vi "Get UUT Error.vi"(8 "error in (no error)":errorcluster, 11 "VISA resource name":refnum<visa-resource-name>) -> (0 "error out":errorcluster, 1 "Error Units":i32, 2 "Value of Error":dbl format="%.4f", 3 "VISA resource name out":refnum<visa-resource-name>)   [LabVIEW 2011, in "Fluke 5XXX Series Multicalibrators.lvlib"]
doc: "This VI returns the UUT error and units computed by the Calibrator after shifting the output with the FL5XMCAL Change Output Value.vi. The UUT error is not computed when editing frequency."
uses:
  Fluke 5XXX Series Multicalibrators.lvlib
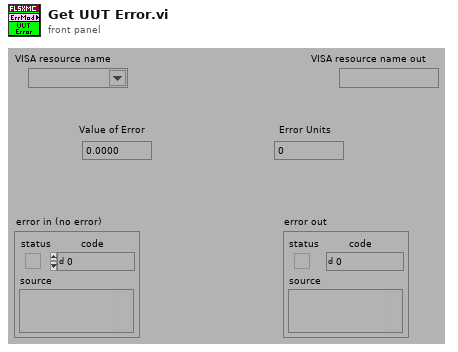
[diagram p1: front panel]
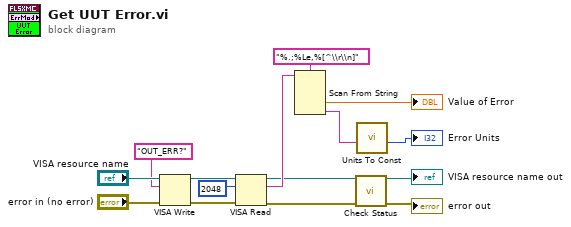
[diagram p0: block diagram]
diagram:
  n1 = VISA Write(VISA resource name="VISA resource name", write buffer="OUT_ERR?", error in (no error)="error in (no error)") -> (VISA resource name out=w13:refnum<visa-resource-name>, error out=w12:errorcluster)  [unwired: 1 out]
  n2 = VISA Read(VISA resource name=w13, byte count=u32 2048 ("byte count (0)"), error in (no error)=w12) -> (VISA resource name out=w2:refnum<visa-resource-name>, read buffer=w11:string, error out=w3:errorcluster)  [unwired: 1 out]
  n3 = Scan From String(format string="%.;%Le,%[^\\r\\n]", input string=w11) -> (output 1=→"Value of Error":dbl, output 2=w1:string)  [unwired: 4 in, 3 out]
  n4 = call "Check Status.vi"("VISA resource name"=w2, "error in (no error)"=w3) -> ("VISA resource name out"=→"VISA resource name out":refnum<visa-resource-name>, "error out"=→"error out":errorcluster)  [unwired: 12 in]
  n5 = call "Units To Const.vi"("Units"=w1) -> ("Const"=→"Error Units":i32)  [unwired: 10 in]
